vi "Configuration dialog.vi"(8 "error in (no error)":errorcluster, 11 "Data in":T3) -> (0 "error out":errorcluster, 2 "Cancelled?":bool=TRUE, 3 "Data out":T3)   [LabVIEW 2020, in "Configuration.lvlib"]
uses:
  Configuration.lvlib
  Config data.ctl
  Support/Accept button.ctl
  Support/Cancel button.ctl
panel:
  in  "Osciloscopio":refnum<visa-resource-name>
  in  "Pitch":dbl=0.025 caption="Paso del tornillo"
  in  "Cancel Button":T1
  in  "OK Button":T2
  in  "Pasos por revolución":dbl=200.0
  in  "DAQ":tag
  # "Avance: 25um/paso\nAvance por revolución: 5mm/rev"
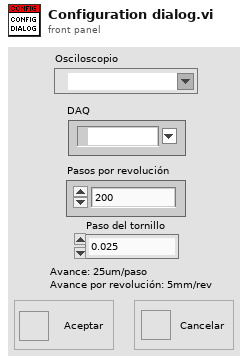
[diagram p1: front panel]
types:
  T1 = typedef "Cancel button.ctl" = bool
  T2 = typedef "Accept button.ctl" = bool
  T3 = typedef "Configuration.lvlib/Config data.ctl" = cluster{"Arduino":string, "Steps per rev":dbl, "Config path":path, "Pitch":dbl, "Osciloscopio":refnum<visa-resource-name>}
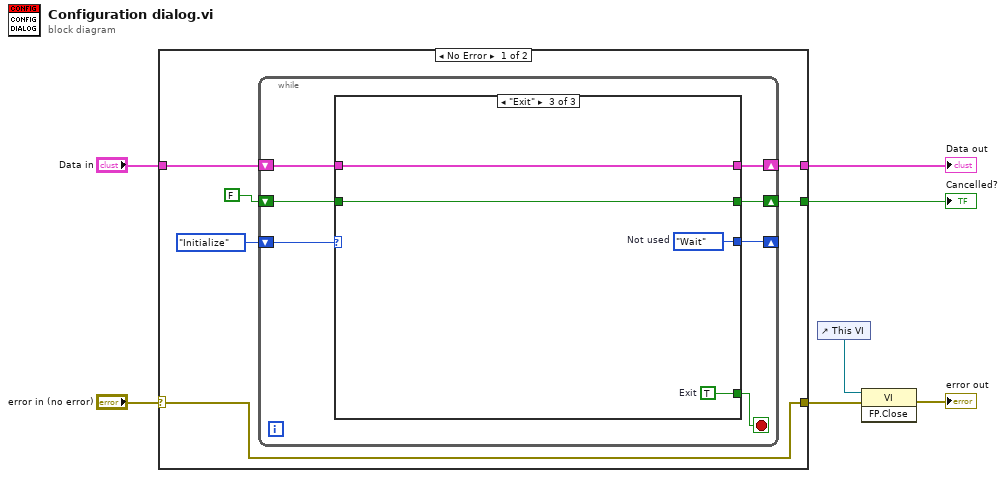
[diagram p0: block diagram]
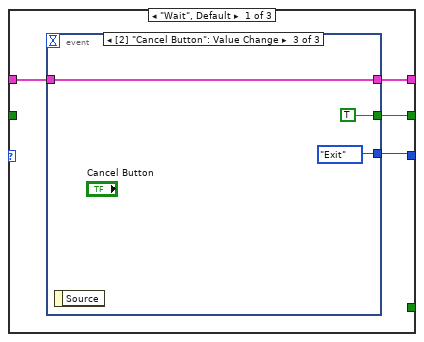
[diagram p2: hidden frame]
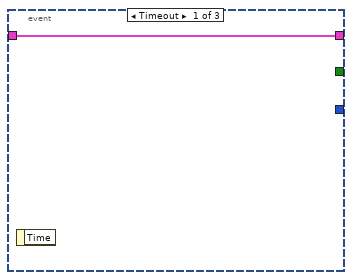
[diagram p3: hidden frame]
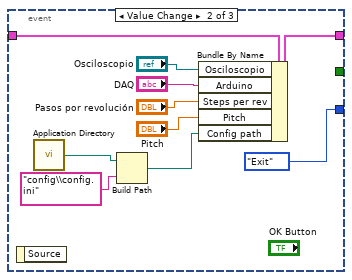
[diagram p4: hidden frame]
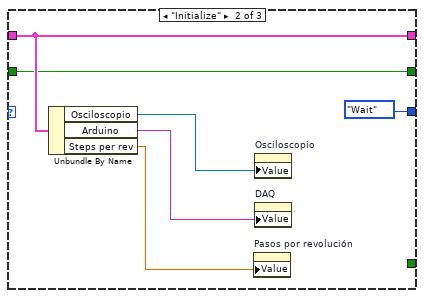
[diagram p5: hidden frame]
diagram:
  n1 = case shown="No Error" "error in (no error)" {
    selector: "error in (no error)" -> [w11 w49]
    tunnel: "Data in" -> [w12 w50]
    tunnel: [w10 w50] -> w6
    tunnel: [w11 w49] -> w3
    tunnel: [w9 _] -> w1
    frame No Error {
      n2 = while {
        shift-right: [w18] -> _
        shift-left: enum16{"Wait", "Initialize", "Exit"}."Initialize" -> [w20]
        shift-right: [w16] -> w10
        shift-left: w12 -> [w17]
        shift-right: [w15] -> w9
        shift-left: FALSE -> [w14]
        stop <- w19 stop-if-true
        n3 = case shown="\"Exit\"" w20 {
          tunnel: [_ _ w48] -> w19
          tunnel: [w22 enum16{"Wait", "Initialize", "Exit"}."Wait" w47] -> w18
          tunnel: w17 -> [w24 w43 w46]
          tunnel: [w23 w43 w46] -> w16
          tunnel: [w21 w39 w45] -> w15
          tunnel: w14 -> [_ w39 w45]
          frame "Wait", Default {
            n4 = event shown="[2] \"Cancel Button\": Value Change" {
              selector: _ -> [_ _ _]
              dyn-events: _ -> [_ _ _]
              timeout: _ -> [_ _ _]
              tunnel: w24 -> [w25 w33 w38]
              tunnel: [w25 w32 w38] -> w23
              tunnel: [_ enum16{"Wait", "Initialize", "Exit"}."Exit" enum16{"Wait", "Initialize", "Exit"}."Exit"] -> w22
              tunnel: [_ _ TRUE] -> w21
              event Timeout {
                n5 = event-data() -> ()  [unwired: 1 in, 1 out]
              }
              event Value Change {
                n6 = event-data() -> ()  [unwired: 1 in, 1 out]
                n7 = call <vilib>:"Application Directory.vi"() -> ("Application Directory"=w28:path)
                n8 = Build Path(base path=w28, name or relative path="config\\config.ini" ("default name")) -> (appended path=w26:path)
                n9 = Bundle By Name(cluster=w33, "Osciloscopio"="Osciloscopio", "Arduino"="DAQ", "Steps per rev"="Pasos por revolución", "Pitch"="Pitch", "Config path"=w26) -> (w32:T3)
              }
              event Value Change {
                n10 = event-data() -> ()  [unwired: 1 in, 1 out]
              }
            }
          }
          frame "Initialize" {
            n11 = Unbundle By Name(w43) -> ("Osciloscopio"=w40:refnum<visa-resource-name>, "Arduino"=w42:string, "Steps per rev"=w41:dbl)
            n12 = property on="Pasos por revolución" class="DigNum (strict)"("Value"=w41) -> ()  [unwired: 2 in, 2 out]
            n13 = property on="Osciloscopio" class="VISAName"("Value"=w40) -> ()  [unwired: 2 in, 2 out]
            n14 = property on="DAQ" class="DAQmxName"("Value"=w42) -> ()  [unwired: 2 in, 2 out]
          }
          frame "Exit" {
            w47 = enum16{"Wait", "Initialize", "Exit"}."Wait"  # Not used
            w48 = TRUE  # Exit
          }
        }
      }
    }
    frame Error {
    }
  }
  "Data out" <- w6
  "Cancelled?" <- w1
  n15 = control-ref of="This VI"() -> (w4:refnum<vi>)
  n16 = invoke class="VI" method="FP.Close"(reference=w4, error in=w3) -> (error out=→"error out":errorcluster)  [unwired: 1 in, 2 out]
